vi "ShooterSpeedRegulateV2 Debug.vi"(11 "Reset Shooter PID":bool) -> (4 "ALL GOOD":bool, 10 "Motor 1 Output":dbl)   [LabVIEW 2012]
uses:
  Robot Global Data.vi
  Max'sToolKit/ConvertVoltageToPercentVbs.vi
panel:
  out "PID Output":dbl
  in  "Shooter Speed":T1(ring)
  in  "Use PID":bool
  out "Waveform Chart":cluster{dbl, "upper limit":dbl, dbl}(graph)
  in  "Feed Foward \nVoltage":dbl format="%_6g"
  in  "PID gains":T2 {"proportional gain (Kp)" format="%_6g"; "integral gain (Ki)" format="%_6g"; "derivative gain (Kd)" format="%_6g"}
  out "Motor Voltage":dbl
  out "Error":dbl
  out "Loop Rate (Hz)":dbl
  out "Array Index":dbl
  out "Wheel 1 RPS":dbl
  in  "W1 Target RPS":dbl
  # "7 Volts are the win for front of pyramid shot"
  # "7 Volts for back of pyramid also"
  # "MAXIMUM POWER for feeeder shot"
  # "64 RPS long 3pt shot"
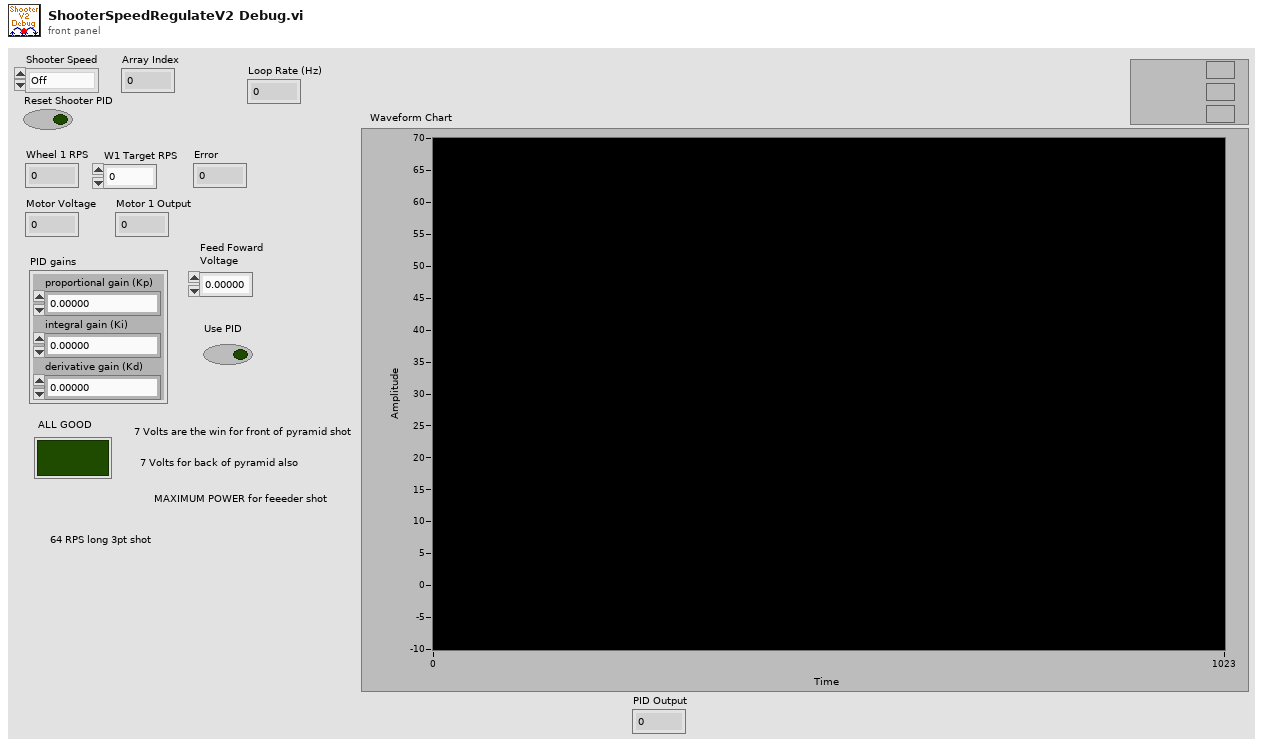
[diagram p1: front panel]
types:
  T1 = enum16{"Off", "Close Pyramid 3pt", "Far Pyramid 3pt", "Feeder Shot"}
  T2 = cluster{"proportional gain (Kp)":dbl, "integral gain (Ki)":dbl, "derivative gain (Kd)":dbl}
  T3 = typedef "WPI_EncoderDevRef.ctl" = cluster{"DevStatus":errorcluster, "EncoderIndex":T4, "CounterIndex":T5, "DistancePerCount":dbl, "Decoding Type":T6}
  T4 = typedef "FPGA_EncoderIdx.ctl" = enum8{"Enc 0", "Enc 1", "Enc 2", "Enc 3", "Invalid"}
  T5 = typedef "FPGA_CounterCtrSystemIndex.ctl" = enum8{"Ctr 0", "Ctr 1", "Ctr 2", "Ctr 3", "Ctr 4", "Ctr 5", "Ctr 6", "Ctr 7", "Invalid"}
  T6 = typedef "WPI_EncoderType.ctl" = enum16{"1x", "2x", "4x"}
  T7 = cluster{"Target Voltage":dbl, "Target Speed":dbl, "Angle Up?":bool}[]
  T8 = cluster{"Target Voltage":dbl, "Target Speed":dbl, "Angle Up?":bool}
  T9 = typedef "WPI_MotorControlDeviceRef.ctl" = cluster{"DeviceStatus":errorcluster, "Type":enum16{"PWM", "CAN"}, "PWM":cluster{"Digital Module":T10, "PWM Channel":T11, "DeadBand":T12}, "CAN":cluster{"Device Number":u8, "Control Mode":T13, "Semaphore":T14, "Max Vout":dbl}, "Invert":bool, "TransformRef":T15, "InvTransformRef":T15}
  T10 = typedef "FPGA_TypedefDigitalModule.ctl" = enum16{"Digital Module 1", "Digital Module 2"}
  T11 = typedef "FPGA_DIOPWMChannel.ctl" = enum8{"PWM 1", "PWM 2", "PWM 3", "PWM 4", "PWM 5", "PWM 6", "PWM 7", "PWM 8", "PWM 9", "PWM 10", "Invalid"}
  T12 = typedef "WPI_PWMDeadband.ctl" = cluster{"Name":string, "maxPositivePwm":i32, "minPositivePwm":i32, "centerPwm":i32, "maxNegativePwm":i32, "minNegativePwm":i32, "angularRange":u16}
  T13 = typedef "WPI_CANJaguar_ControlMode.ctl" = enum8{"Percent VBus", "Current", "Speed", "Position", "Voltage"}
  T14 = typedef "Semaphore RefNum" = refnum<k1>
  T15 = typedef "WPI_PWMTransform_ConPane.ctl" = refnum<vi>
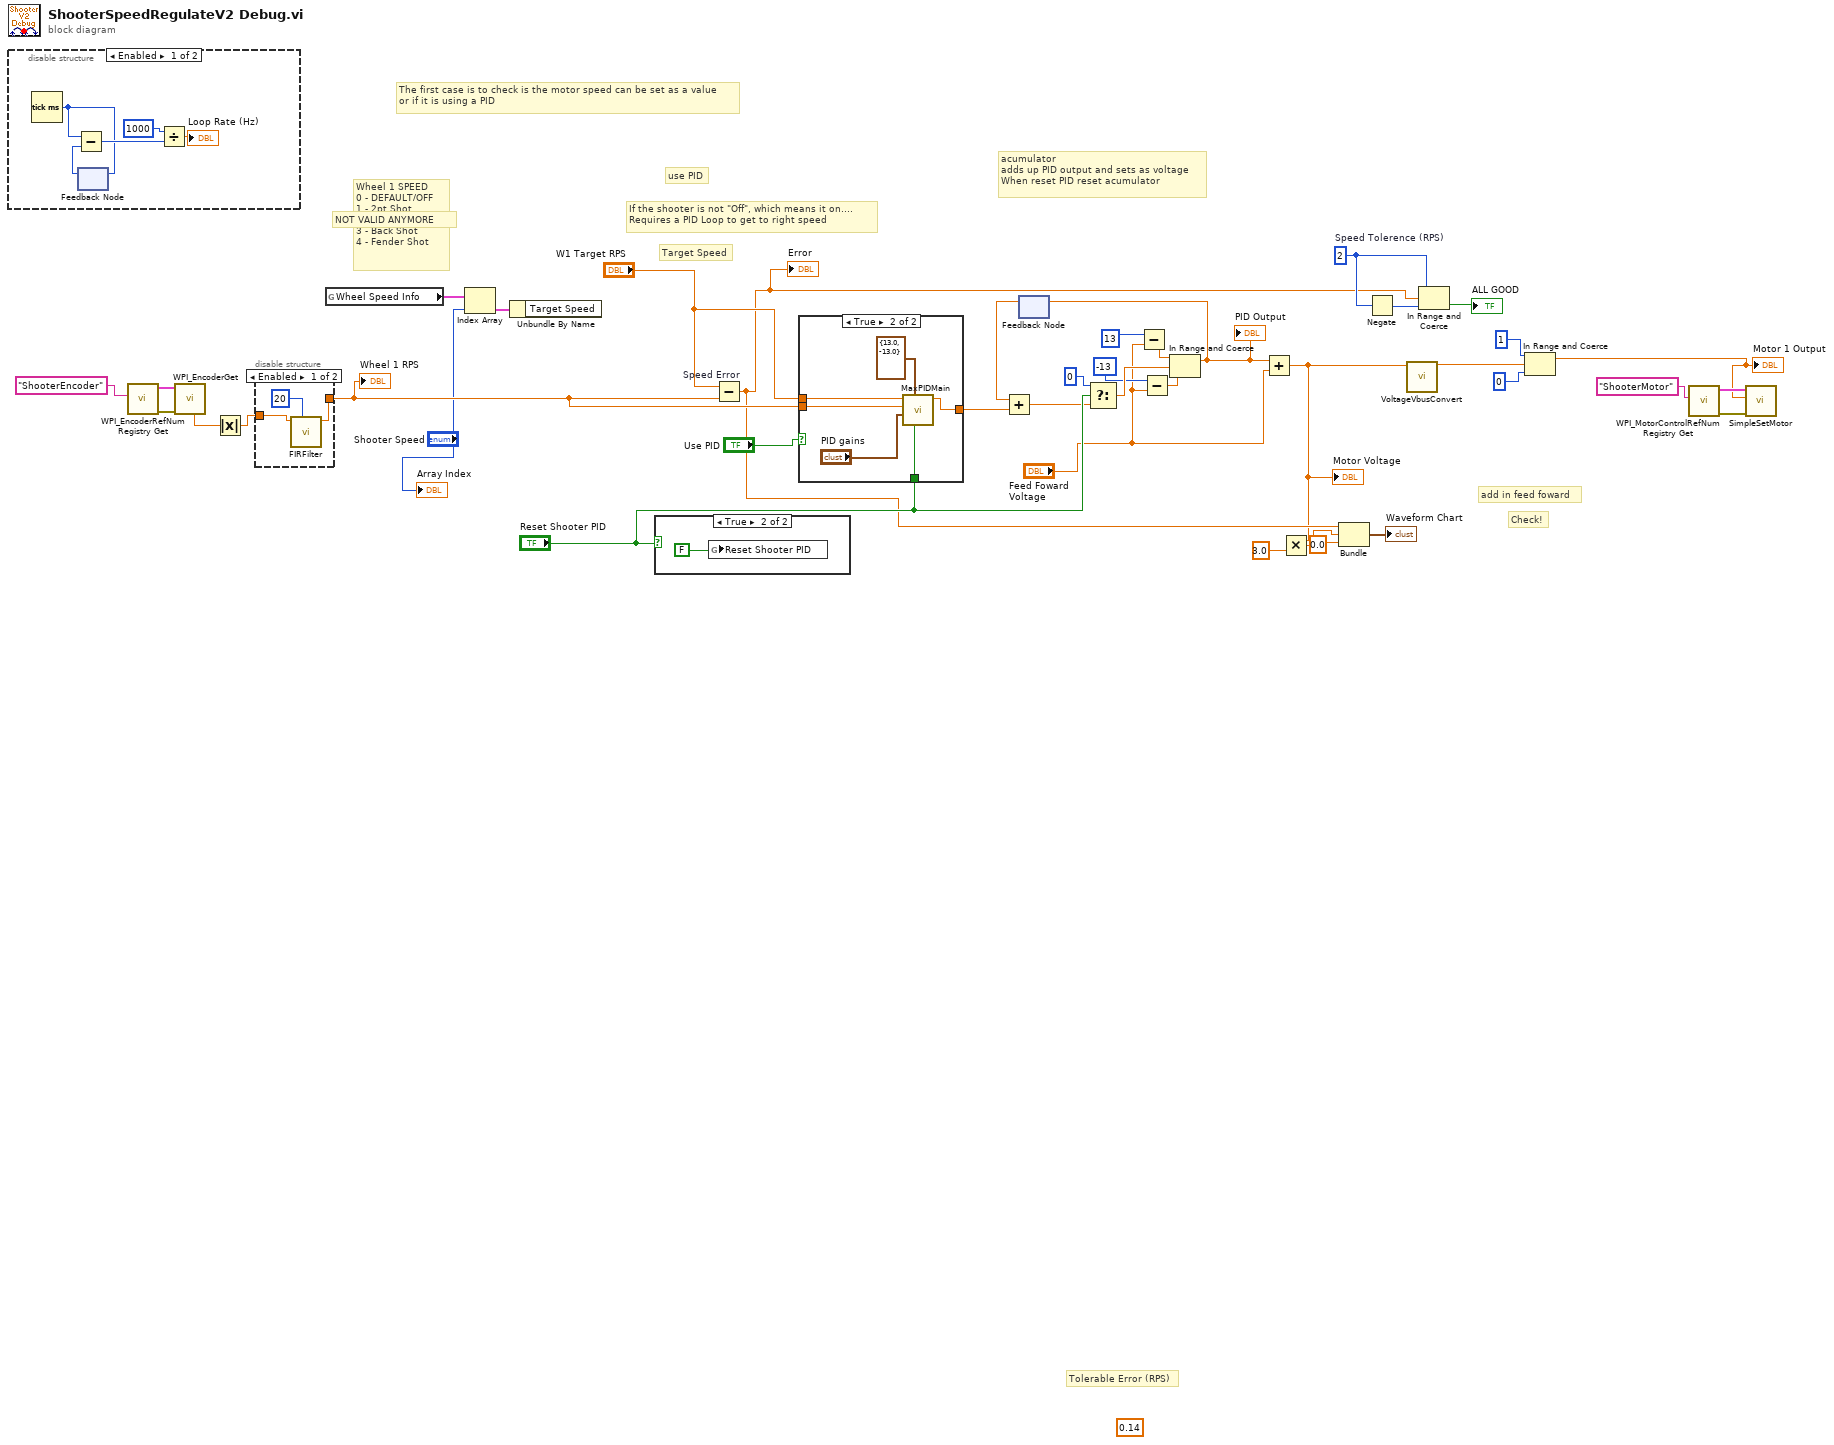
[diagram p0: block diagram]
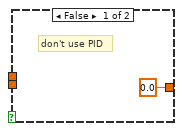
[diagram p2: hidden frame]
diagram:
  w26 = 2  # Speed Tolerence (RPS)
  (unwired) 0.14
  # "Check!"
  # "add in feed foward"
  # "acumulator\nadds up PID output and sets as voltage\nWhen reset PID reset acumulator"
  # "Target Speed"
  # "If the shooter is not \"Off\", which means it on....\nRequires a PID Loop to get to right speed"
  # "use PID"
  # "NOT VALID ANYMORE"
  # "The first case is to check is the motor speed can be set as a value\nor if it is using a PID"
  # "Tolerable Error (RPS)"
  # "Wheel 1 SPEED\n0 - DEFAULT/OFF\n1 - 2pt Shot\n2 - 3pt Key Shot\n3 - Back Shot\n4 - Fender Shot"
  n1 = disable-structure shown="Enabled" {
    frame Enabled {
      n2 = Tick Count (ms)() -> (millisecond timer value=w40:u32)
      n3 = feedback #1() -> (w41:u32)  [unwired: 1 in]
      n4 = Subtract(x=w40, y=w41) -> (x-y=w43:u32)
      n5 = feedback-in #1(w40) -> ()
      n6 = Divide(x=1000, y=w43) -> (x/y=→"Loop Rate (Hz)":dbl)
    }
    frame Disabled {
    }
  }
  n7 = call <vilib>:"WPI_EncoderRefNum Registry Get.vi"("refnum name"="ShooterEncoder") -> ("error out"=w33:errorcluster, "EncoderDevRef"=w34:T3)  [unwired: 9 in]
  n8 = call <vilib>:"WPI_EncoderGet.vi"("error in (no error)"=w33, "EncoderDevRef"=w34) -> ("Rate"=w30:dbl)  [unwired: 4 in, 5 out]
  n9 = Absolute Value(x=w30) -> (abs(x)=w29:dbl)
  n10 = disable-structure shown="Enabled" {
    disable-tunnel: [w47 w48] -> w32
    disable-tunnel: w29 -> [w46 w48]
    frame Enabled {
      n11 = call "FIRFilter.vi"("Filter Size"=i8 20, "Input"=w46) -> ("Output"=w47:dbl)  [unwired: 9 in]
    }
    frame Disabled {
    }
  }
  "Wheel 1 RPS" <- w32
  n12 = global read "Robot Global Data.vi" "Wheel Speed Info"() -> (w31:T7)
  n13 = Index Array(array=w31, index="Shooter Speed") -> (element=w9:T8)
  n14 = Unbundle By Name(w9) -> ()  [unwired: 1 out]
  n15 = case shown="True" "Reset Shooter PID" {
    frame False {
    }
    frame True {
      n16 = global write "Robot Global Data.vi" "Reset Shooter PID"(FALSE) -> ()
    }
  }
  n17 = Subtract "Speed Error"(x="W1 Target RPS", y=w32) -> (x-y=w7:dbl)
  "Error" <- w7
  n18 = case shown="True" "Use PID" {
    tunnel: w32 -> [_ w56]
    tunnel: "Reset Shooter PID" -> [_ w55]
    tunnel: "W1 Target RPS" -> [_ w52]
    tunnel: [0.0 ("output") w51] -> w23
    frame False {
      # "don't use PID"
    }
    frame True {
      n19 = call "MaxPIDMain.vi"("Reset"=w55, "Output Range"=cluster{"output high":dbl, "output low":dbl} {"output high"=13.0, "output low"=-13.0} ("output range"), "PID gains"="PID gains", "process variable"=w56, "setpoint"=w52) -> ("Output"=w51:dbl)  [unwired: 5 in, 1 out]
    }
  }
  n20 = feedback #2() -> (w24:dbl)  [unwired: 1 in]
  n21 = Add(x=w24, y=w23) -> (x+y=w18:dbl)
  n22 = Select(t=0, s="Reset Shooter PID", f=w18) -> (s? t:f=w22:dbl)
  n23 = Subtract(x=13 ("upper limit"), y="Feed Foward \nVoltage") -> (x-y=w16:dbl)
  n24 = Subtract(x=-13 ("upper limit"), y="Feed Foward \nVoltage") -> (x-y=w4:dbl)
  n25 = In Range and Coerce(upper limit=w16, x=w22, lower limit=w4) -> (coerced(x)=w15:dbl)  [unwired: 1 out]
  "PID Output" <- w15
  n26 = feedback-in #2(w15) -> ()
  n27 = Add(x=w15, y="Feed Foward \nVoltage") -> (x+y=w3:dbl)
  "Motor Voltage" <- w3
  n28 = Multiply(x=w3, y=3.0) -> (x*y=w2:dbl)
  n29 = Bundle(w7, w2, 0.0) -> (→"Waveform Chart":cluster{dbl, dbl, dbl})  [unwired: 1 in]
  n30 = Negate(x=w26) -> (-x=w36:i32)
  n31 = call-poly "VoltageVbusConvert.vi"("Voltage"=w3) -> ("Vbus"=w11:dbl)  [unwired: 10 in]
  n32 = In Range and Coerce(upper limit=w26, x=w7, lower limit=w36) -> (In Range?=→"ALL GOOD":bool)  [unwired: 1 out]
  n33 = In Range and Coerce(upper limit=1, x=w11, lower limit=0 ("upper limit")) -> (coerced(x)=w13:dbl)  [unwired: 1 out]
  "Motor 1 Output" <- w13
  n34 = call <vilib>:"WPI_MotorControlRefNum Registry Get.vi"("refnum name"="ShooterMotor") -> ("error out"=w37:errorcluster, "MotorControlDevRef"=w38:T9)  [unwired: 9 in]
  n35 = call "SimpleSetMotor.vi"("error in (no error)"=w37, "Output"=w13, "MotorControlDevRef"=w38) -> ()  [unwired: 7 in, 2 out]
  "Array Index" <- "Shooter Speed"
